vi "PD500 - PWM test.vi"(7 "Board Selector":T1, 9 "HMP4040_IN":refnum<visa-resource-name>, 10 "Message IN":string=" ", 11 "HMP4040 Channel Settings":T2={"CH1 Voltage"=24.0, "CH1 Current"=1.0, "CH1 Output"=TRUE, "CH2 Voltage"=24.0, "CH2 Current"=1.0, "CH2 Output"=TRUE, "CH3 Voltage"=24.0, "CH3 Current"=1.0, "CH3 Output"=TRUE, "CH4 Voltage"=24.0, "CH4 Current"=1.0, "CH4 Output"=TRUE, "Master Output"=TRUE} {"CH4 Current" format="%.3f"; "CH4 Voltage" format="%.3f"; "CH3 Current" format="%.3f"; "CH3 Voltage" format="%.3f"; "CH2 Current" format="%.3f"; "CH2 Voltage" format="%.3f"; "CH1 Current" format="%.3f"; "CH1 Voltage" format="%.3f"}) -> (0 "error out":errorcluster, 1 "Result (bool)":bool, 2 "Message OUT":string, 3 "ControlBoard OUT":refnum<visa-resource-name>)   [LabVIEW 2022 SP3]
uses:
  HMP4000 Communication/HMP4040_ChannelControl.ctl
  Serial Board Com/Board Select.ctl
  <vilib>/DAQmx/read.llb/DAQmx Read (Analog 1D Wfm NChan NSamp).vi
  <vilib>/DAQmx/miscellaneous.llb/DAQmx Fill In Error Info.vi
panel:
  in  "error in (no error) 2":errorcluster
  out "Duty Cycle VISA Write":string[](array[string])
  out "Duty Cycles Measured":dbl[][](array[numeric])
  out "Analysis Leg":i32
  in  "Debug Mode":bool
  out "Waveforms":T3
  out "Active Leg":i32
  out "Result (color)":u32(colorbox)
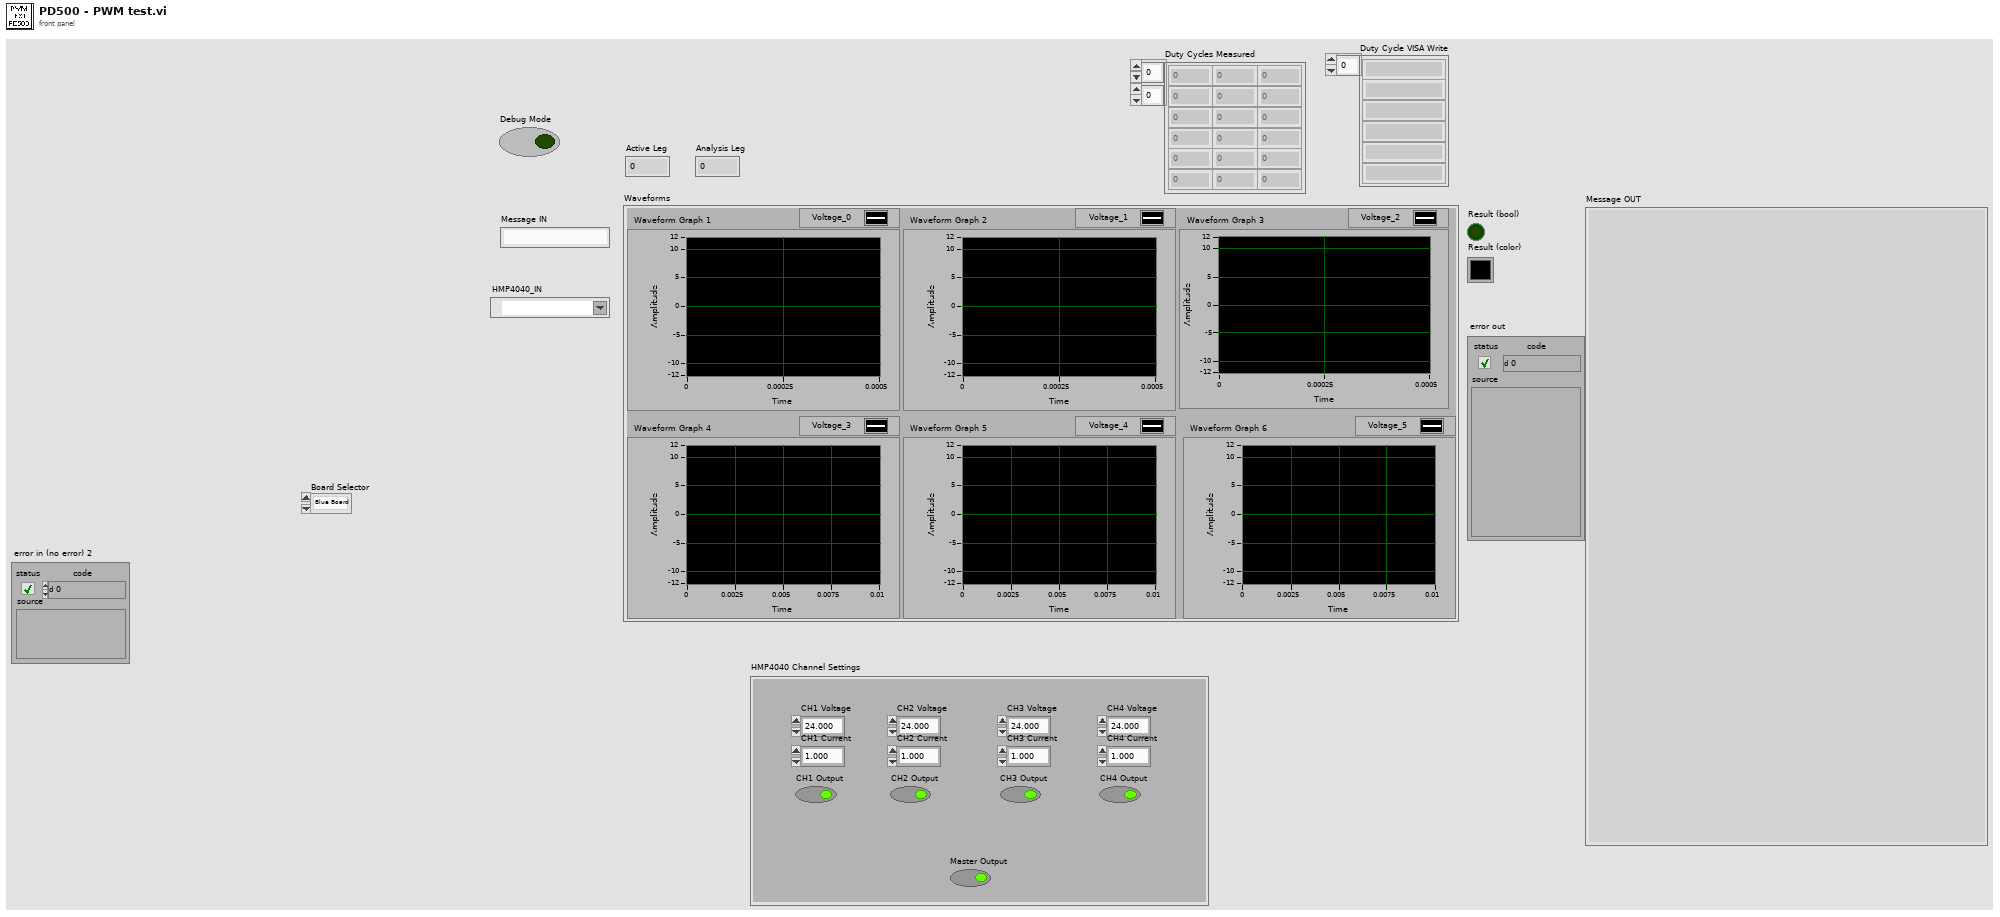
[diagram p1: front panel]
types:
  T1 = typedef "Board Select.ctl" = enum16{"Blue Board", "Green Board"}
  T2 = typedef "HMP4040_ChannelControl.ctl" = cluster{"CH1 Voltage":dbl, "CH1 Current":dbl, "CH1 Output":bool, "CH2 Voltage":dbl, "CH2 Current":dbl, "CH2 Output":bool, "CH3 Voltage":dbl, "CH3 Current":dbl, "CH3 Output":bool, "CH4 Voltage":dbl, "CH4 Current":dbl, "CH4 Output":bool, "Master Output":bool}
  T3 = cluster{"Waveform Graph 1":waveform(dbl), "Waveform Graph 2":waveform(dbl), "Waveform Graph 3":waveform(dbl), "Waveform Graph 4":waveform(dbl), "Waveform Graph 5":waveform(dbl), "Waveform Graph 6":waveform(dbl)}
  T4 = cluster{"data[0]":waveform(dbl), "data[1]":waveform(dbl), "data[2]":waveform(dbl), "data[3]":waveform(dbl), "data[4]":waveform(dbl), "data[5]":waveform(dbl)}
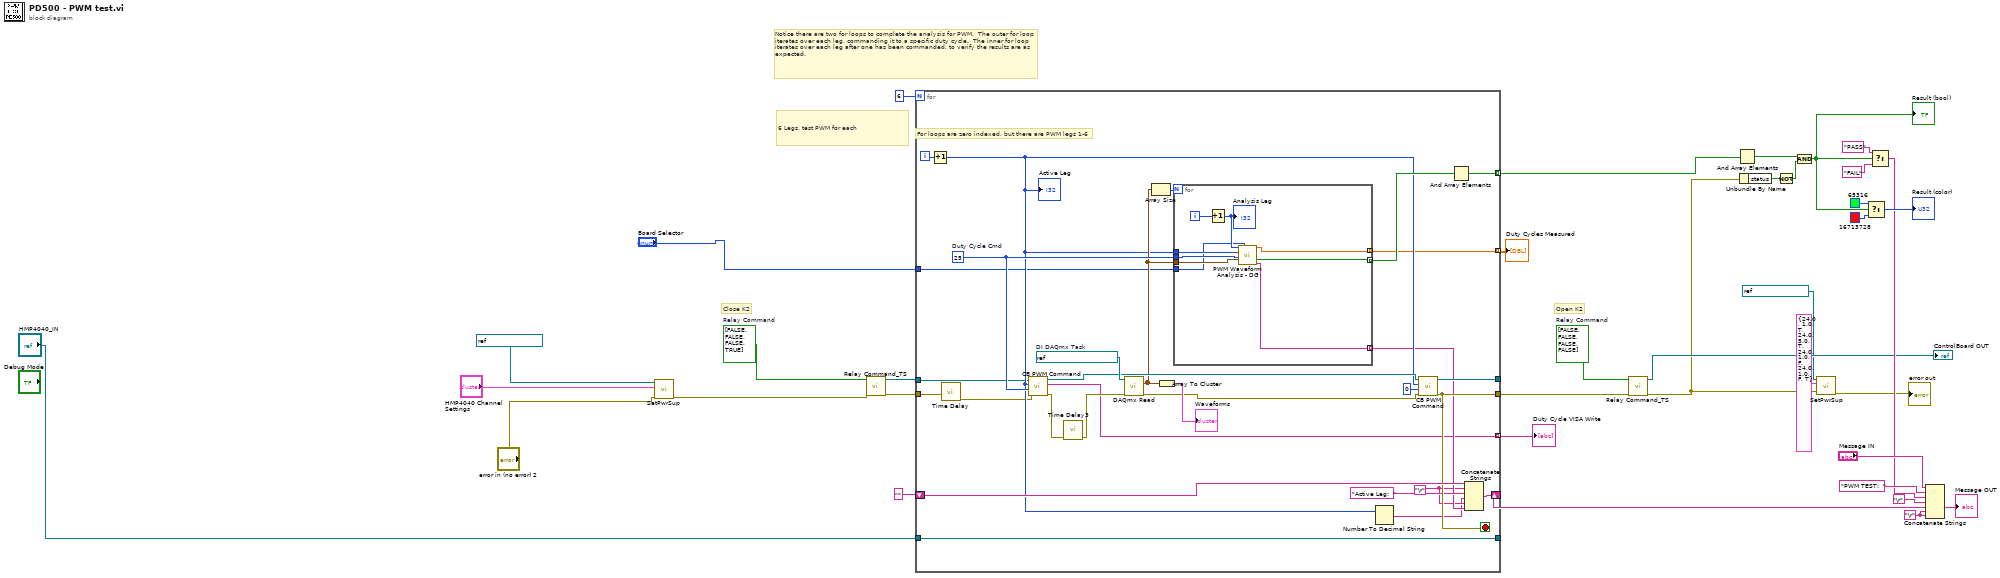
[diagram p0: block diagram]
diagram:
  w11 = bool[] [FALSE, FALSE, FALSE, TRUE]  # Relay Command
  w1 = bool[] [FALSE, FALSE, FALSE, FALSE]  # Relay Command
  w26 = "\r"
  # "Close K2"
  # "Open K2"
  # "Notice there are two for loops to complete the analysis for PWM.  The outer for loop iterates over each leg, commanding it to a specific duty cycle.  The inner for loop iterates over each leg after one has been commanded, to verify the results are as expected."
  # "6 Legs, test PWM for each"
  n1 = call "SetPwrSup.vi"("error in (no error)"="error in (no error) 2", "HMP4040 Channel Settings"="HMP4040 Channel Settings", "HMP4040 IN"=refnum<visa-resource-name> "HMP4040_FTS2" ("VISA resource name")) -> ("error out"=w7:errorcluster)  [unwired: 7 in, 1 out]
  n2 = call "Relay Command_TS.vi"("error in (no error)"=w7, "Relay Command"=w11) -> ("error out"=w14:errorcluster, "VISA Refnum out"=w16:refnum<visa-resource-name>)  [unwired: 8 in]
  n3 = for {
    N: 6 -> [_]
    tunnel: [w66] -> w37 mode=indexing
    shift-right: [w64] -> w24
    shift-left: "" -> [w63]
    tunnel: [w58] -> _
    tunnel: "HMP4040_IN" -> [w58]
    tunnel: [w57] -> w18
    tunnel: [w52] -> _
    tunnel: w14 -> [w40]
    tunnel: w16 -> [w46]
    tunnel: [w43] -> w13 mode=indexing
    tunnel: [w42] -> w12 mode=indexing
    tunnel: "Board Selector" -> [w41]
    i -> [w59]
    stop <- w57 stop-if-true
    w48 = "\r"
    w60 = 25  # Duty Cycle Cmd
    w65 = refnum<k21> "FTS2_PWMInput_DG"  # DI DAQmx Task
    # "For loops are zero indexed, but there are PWM legs 1-6"
    n4 = Increment(x=w59) -> (x+1=w50:i32)
    "Active Leg" <- w50
    n5 = call "Time Delay"("error in (no error)"=w40) -> ("error out"=w39:errorcluster)  [unwired: 10 in]
    n6 = call "CB PWM Command.vi"("error in (no error)"=w39, "Duty Cycle"=w60, "Leg"=w50, "VISA Refnum in"=w46) -> ("error out"=w45:errorcluster, "read buffer"=w42:string, "VISA Refnum out"=w61:refnum<visa-resource-name>)  [unwired: 5 in]
    n7 = call "Time Delay3"("error in (no error)"=w45) -> ("error out"=w44:errorcluster)  [unwired: 10 in]
    n8 = call-poly <vilib>:"DAQmx Read.vi"("task/channels in"=w65, "error in"=w44) -> ("data"=w53:waveform(dbl)[], "error out"=w38:errorcluster)  [unwired: 11 in, 1 out]
    n9 = Array Size(array=w53) -> (size(s)=w54:i32)
    n10 = Array To Cluster(array=w53) -> (cluster=→"Waveforms":T4)
    n11 = for {
      N: w54 -> [_]
      tunnel: w60 -> [w75]
      tunnel: w53 -> [w74]
      tunnel: w50 -> [w73]
      tunnel: [w70] -> w55 mode=indexing
      tunnel: [w69] -> w49 mode=indexing
      tunnel: [w68] -> w43 mode=indexing
      tunnel: w41 -> [w67]
      i -> [w72]
      n12 = Increment(x=w72) -> (x+1=w71:i32)
      "Analysis Leg" <- w71
      n13 = call "PWM Waveform Analysis - DG.vi"("Analysis Leg"=w71, "Board Selector"=w67, "Active Leg"=w73, "Duty Cycle"=w75, "Waveform"=w74) -> ("Active Leg Actual Duty"=w68:dbl, "Result (Boolean)"=w70:bool, "Message"=w69:string)  [unwired: 8 in]
    }
    n14 = Number To Decimal String(number=w50) -> (decimal integer string=w47:string)  [unwired: 1 in]
    n15 = call "CB PWM Command.vi"("error in (no error)"=w38, "Duty Cycle"=0, "Leg"=w50, "VISA Refnum in"=w61) -> ("error out"=w57:errorcluster, "VISA Refnum out"=w52:refnum<visa-resource-name>)  [unwired: 5 in, 1 out]
    n16 = And Array Elements(Boolean array=w55) -> (logical AND=w66:bool)
    n17 = Concatenate Strings(w63, w48, "Active Leg:  ", w47, w48, w49) -> (w64:string)
  }
  "Duty Cycles Measured" <- w13
  "Duty Cycle VISA Write" <- w12
  n18 = call "Relay Command_TS.vi"("error in (no error)"=w18, "Relay Command"=w1) -> ("error out"=w4:errorcluster, "VISA Refnum out"=→"ControlBoard OUT":refnum<visa-resource-name>)  [unwired: 8 in]
  n19 = And Array Elements(Boolean array=w37) -> (logical AND=w27:bool)
  n20 = Unbundle By Name(w4) -> ("status"=w30:bool)
  n21 = Not(x=w30) -> (.not. x?=w29:bool)
  n22 = And(x=w27, y=w29) -> (x .and. y?=w28:bool)
  "Result (bool)" <- w28
  n23 = call "SetPwrSup.vi"("error in (no error)"=w4, "HMP4040 Channel Settings"=T2 {"CH1 Voltage"=24.0, "CH1 Current"=1.0, "CH1 Output"=TRUE, "CH2 Voltage"=24.0, "CH2 Current"=5.0, "CH2 Output"=TRUE, "CH3 Voltage"=24.0, "CH3 Current"=1.0, "CH3 Output"=FALSE, "CH4 Voltage"=24.0, "CH4 Current"=1.0, "CH4 Output"=FALSE, "Master Output"=TRUE}, "HMP4040 IN"=refnum<visa-resource-name> "HMP4040_FTS2" ("VISA resource name")) -> ("error out"=→"error out":errorcluster)  [unwired: 7 in, 1 out]
  n24 = Select(t=u32 65316 ("Result (color)"), s=w28, f=u32 16713728 ("Result (color)")) -> (s? t:f=→"Result (color)":u32)
  n25 = Select(t="PASS", s=w28, f="FAIL") -> (s? t:f=w19:string)
  n26 = Concatenate Strings("Message IN", "PWM TEST:  ", w19, "\r", w24, w26, w26) -> (→"Message OUT":string)
